vi "Read MonoState.vi"(8 "error in (no error)":errorcluster, 11 "Monochromator in":refnum<class "Monochromator.lvclass">) -> (0 "error out":errorcluster, 2 "MonoState.lvclass":refnum<class "MonoState.lvclass">, 3 "Monochromator out":refnum<class "Monochromator.lvclass">)   [LabVIEW 2016, in "Monochromator.lvclass"]
uses:
  Monochromator.lvclass
  MonoStates/MonoState/MonoState.lvclass
  Monochromator.lvclass/Monochromator.ctl
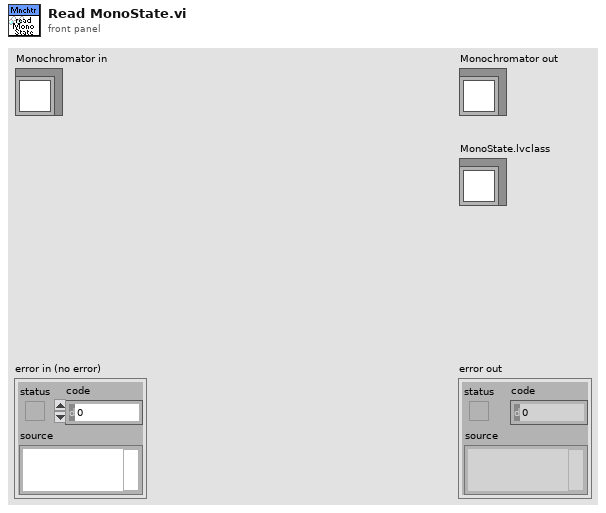
[diagram p1: front panel]
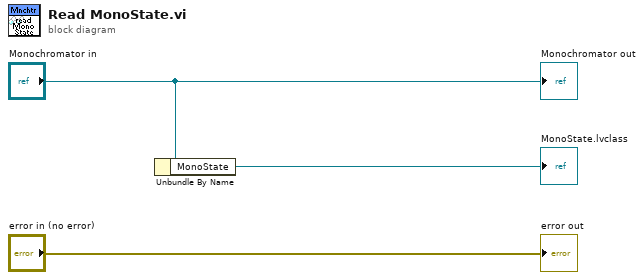
[diagram p0: block diagram]
diagram:
  n1 = Unbundle By Name("Monochromator in") -> ("MonoState"=→"MonoState.lvclass":refnum<class "MonoState.lvclass">)
  "error out" <- "error in (no error)"
  "Monochromator out" <- "Monochromator in"
